vi "Thor_MoveRelative.vi"(5 "Step Size":dbl, 7 "Direction":i32(ring)=1 items=["Forward"=1, "Backward"=2], 8 "error in":errorcluster, 10 "Device In":T1, 11 "KCubeServoControl In":T2) -> (0 "error out":errorcluster, 2 "Device Out":T1, 3 "KCubeServoControl out":T2)   [LabVIEW 2020]
uses:
  Thor_KCubeServoDCRef.ctl
  E:/Norway Project/All Hardware/New Microscope/LabVIEW/ThorLabs/Thorlabs.MotionControl.Controls.dll
  Thorlabs.MotionControl.Controls.dll
  Thor_DeviceRef.ctl
  E:/Norway Project/All Hardware/New Microscope/LabVIEW/ThorLabs/ThorLabs.MotionControl.KCube.DCServoCLI.dll
  ThorLabs.MotionControl.KCube.DCServoCLI.dll
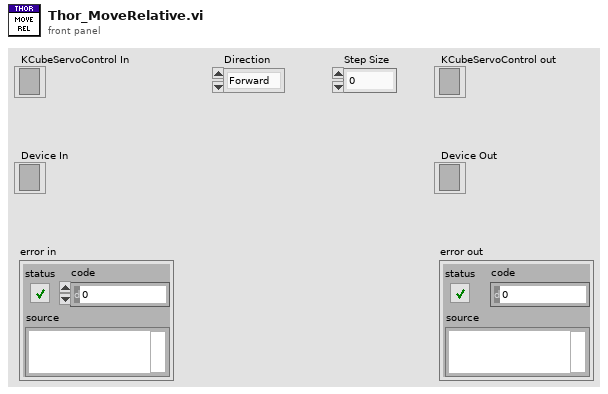
[diagram p1: front panel]
types:
  T1 = typedef "Thor_DeviceRef.ctl" = refnum<k24>
  T2 = typedef "Thor_KCubeServoDCRef.ctl" = refnum<k24>
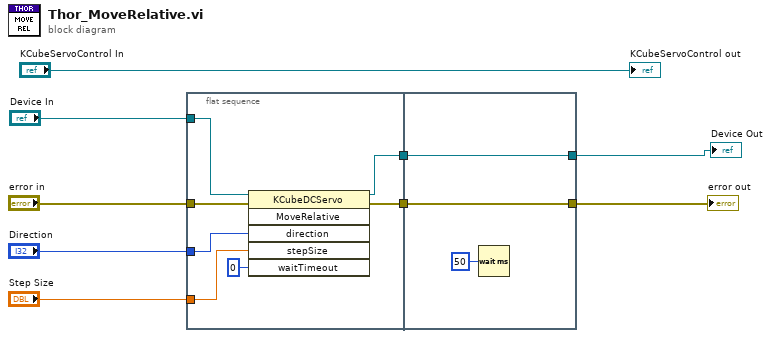
[diagram p0: block diagram]
diagram:
  n1 = flat-sequence {
    tunnel: "error in" -> [w15]
    tunnel: "Step Size" -> [w13]
    tunnel: "Direction" -> [w12]
    tunnel: "Device In" -> [w11]
    tunnel: [w16] -> w2
    tunnel: [w10] -> w1
    tunnel: [w18] -> w3
    tunnel: [w19] -> w9
    tunnel: w2 -> [w19]
    tunnel: w1 -> [w18]
    frame #0 {
      n2 = invoke class="KCubeDCServo" method="MoveRelative"(reference=w11, error in=w15, "direction"=w12, "stepSize"=w13, "waitTimeout"=0) -> (reference out=w10:T1, error out=w16:errorcluster)  [unwired: 1 in, 4 out]
    }
    frame #1 {
      n3 = Wait (ms)(milliseconds to wait=u32 50) -> ()  [unwired: 1 out]
    }
  }
  "error out" <- w9
  "KCubeServoControl out" <- "KCubeServoControl In"
  "Device Out" <- w3
